vi "TDMS_Initialize.vi"(9 "Channel IDs":string[](array[string]), 10 "TDMS Name":string, 11 "Log to USB?":bool=TRUE) -> (3 "TDMS Cluster":T1)   [LabVIEW 2016]
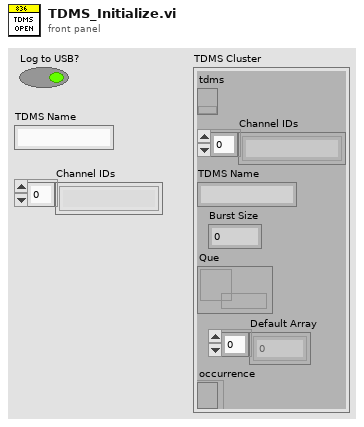
[diagram p1: front panel]
types:
  T1 = cluster{"tdms":refnum<k34>, "Channel IDs":string[], "TDMS Name":string, "Burst Size":i32, "Que":refnum<k33>, "Default Array":dbl[], "occurrence":refnum<k4>}
  T2 = enum16{"open", "open or create", "create or replace", "create", "open (read-only)"}
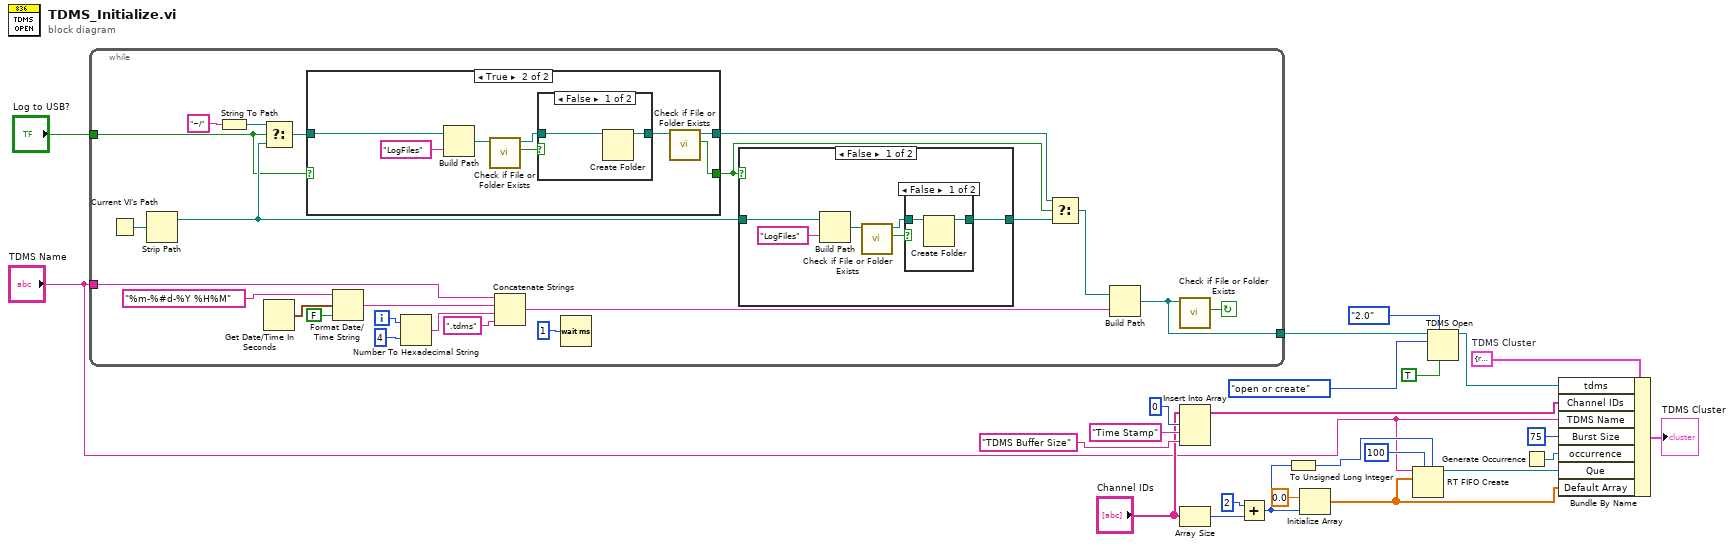
[diagram p0: block diagram]
diagram:
  w22 = T1 {"tdms"=refnum, "Channel IDs"=[], "TDMS Name"="", "Burst Size"=0, "Que"=refnum, "Default Array"=[], "occurrence"=refnum}  # TDMS Cluster
  n1 = while {
    tunnel: [w37] -> w12
    tunnel: "Log to USB?" -> [w26]
    tunnel: "TDMS Name" -> [w25]
    i -> [w41]
    stop <- w38 continue-if-true
    n2 = Current VI's Path() -> (path=w36:path)
    n3 = Strip Path(path=w36) -> (stripped path=w30:path)  [unwired: 1 out]
    n4 = String To Path(string="~/") -> (path=w34:path)
    n5 = Select(t=w34, s=w26, f=w30) -> (s? t:f=w35:path)
    n6 = Get Date/Time In Seconds() -> (seconds since 1Jan1904=w43:timestamp)
    n7 = case shown="True" w26 {
      selector: w26 -> [w49 _]
      tunnel: w35 -> [w48 w54]
      tunnel: [w48 w51] -> w32
      tunnel: [w49 w50] -> w29
      frame False {
      }
      frame True {
        n8 = Build Path(base path=w54, name or relative path="LogFiles") -> (appended path=w53:path)
        n9 = call <vilib>:"Check if File or Folder Exists.vi"("path"=w53) -> ("file or folder exists?"=w57:bool, "dup path"=w56:path)  [unwired: 8 in, 1 out]
        n10 = case shown="False" w57 {
          tunnel: [w59 w60] -> w52
          tunnel: w56 -> [w58 w60]
          frame False {
            n11 = Create Folder(path (use dialog)=w58) -> (created path=w59:path)  [unwired: 2 in, 2 out]
          }
          frame True {
          }
        }
        n12 = call <vilib>:"Check if File or Folder Exists.vi"("path"=w52) -> ("file or folder exists?"=w50:bool, "dup path"=w51:path)  [unwired: 8 in, 1 out]
      }
    }
    n13 = Format Date/Time String(time format string (%c)="%m-%#d-%Y %H%M", seconds (now)=w43, UTC format=FALSE) -> (date/time string=w46:string)
    n14 = Number To Hexadecimal String(1:i16 4 ("width (-)"), 2:w41) -> (0:w39:string)
    n15 = Concatenate Strings(w25, w46, w39, ".tdms" ("string")) -> (w47:string)
    n16 = Wait (ms)(milliseconds to wait=u32 1 ("millisecond multiple")) -> ()  [unwired: 1 out]
    n17 = case shown="False" w29 {
      tunnel: w30 -> [w65 w70]
      tunnel: [w61 w70] -> w28
      frame False {
        n18 = Build Path(base path=w65, name or relative path="LogFiles") -> (appended path=w62:path)
        n19 = call <vilib>:"Check if File or Folder Exists.vi"("path"=w62) -> ("file or folder exists?"=w63:bool, "dup path"=w64:path)  [unwired: 8 in, 1 out]
        n20 = case shown="False" w63 {
          tunnel: [w68 w69] -> w61
          tunnel: w64 -> [w67 w69]
          frame False {
            n21 = Create Folder(path (use dialog)=w67) -> (created path=w68:path)  [unwired: 2 in, 2 out]
          }
          frame True {
          }
        }
      }
      frame True {
      }
    }
    n22 = Select(t=w32, s=w29, f=w28) -> (s? t:f=w31:path)
    n23 = Build Path(base path=w31, name or relative path=w47) -> (appended path=w37:path)
    n24 = call <vilib>:"Check if File or Folder Exists.vi"("path"=w37) -> ("file or folder exists?"=w38:bool)  [unwired: 8 in, 2 out]
  }
  n25 = Insert Into Array(array="Channel IDs", index=0, new element #1="Time Stamp" ("new element/subarray"), new element #2="TDMS Buffer Size" ("new element/subarray")) -> (w2:string[])
  n26 = Array Size(array="Channel IDs") -> (size(s)=w11:i32)
  n27 = Add(x=2, y=w11) -> (x+y=w10:i32)
  n28 = To Unsigned Long Integer(number=w10) -> (unsigned 32bit integer=w9:u32)
  n29 = Initialize Array(0.0 ("element"), w10) -> (w18:dbl[])
  n30 = RT FIFO Create(0:"TDMS Name", 1:w18, 4:u32 100 ("size (10)"), 6:w9) -> (8:w19:refnum<k33>)  [unwired: 4 in, 2 out]
  n31 = TDMS Open(6:TRUE ("disable buffering? (T)"), 7:enum16{"1.0", "2.0"}."2.0" ("file format version (2.0)"), 10:T2."open or create" ("operation (0:open)"), 11:w12) -> (3:w21:refnum<k34>)  [unwired: 3 in, 1 out]
  n32 = Generate Occurrence() -> (w8:refnum<k4>)
  n33 = Bundle By Name(cluster=w22, "tdms"=w21, "Channel IDs"=w2, "TDMS Name"="TDMS Name", "Burst Size"=75 ("y"), "occurrence"=w8, "Que"=w19, "Default Array"=w18) -> (→"TDMS Cluster":T1)
